vi "Write stateFactory.vi"(10 "stateFactory":refnum<class "IStateFactory.lvclass">, 11 "Model in":refnum<class "Model.lvclass">) -> (3 "Model out":refnum<class "Model.lvclass">)   [LabVIEW 2013, in "Model.lvclass"]
uses:
  Model.lvclass
  IStateFactory/IStateFactory.lvclass
  Model.lvclass/Model.ctl
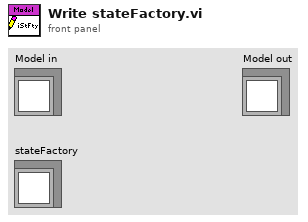
[diagram p1: front panel]
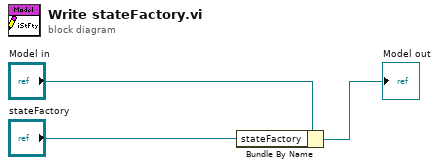
[diagram p0: block diagram]
diagram:
  n1 = Bundle By Name(cluster="Model in", "stateFactory"="stateFactory") -> (→"Model out":refnum<class "Model.lvclass">)
